vi "AudioTest.Parse SoundCheck Data Log TXT File.vi"(6 "Lim Center at Average(f), Float at center":bool, 8 "error in":errorcluster, 9 "Start_End":dbl[](array[numeric])=[500.0, 20000.0], 10 "Config Folder":path=path "C:/MTE/Audio Test/Config", 11 "SoundCheck Data File":path) -> (0 "error out":errorcluster, 1 "Meas Rslt":T3[](array[typedef]) {"Status" items=["LOG", "PASS", "FAIL", "ERROR"]}, 2 "Graph Names":string[](array[string]), 3 "Graphs":T5[](array[typedef]))   [LabVIEW 2018]
uses:
  TypeDefs/AudioTest.Analysis Data Record.ctl
  Common/Utils/Results/Result.Measurement Item.ctl
  Common/Utils/Results/Result.Measurement and Attribute Item Status.ctl
  TypeDefs/AudioTest.Graph Definitions.ctl
  TypeDefs/AudioTest.Result Plot Data.ctl
  Common/Utils/Errors/Error.Error Code List.ctl
  <vilib>/KATE/Files/File Utils.lvlib
panel:
  out "LimitPlots":T1[](array[typedef])
  out "Graph Defs":T2[](array[typedef])
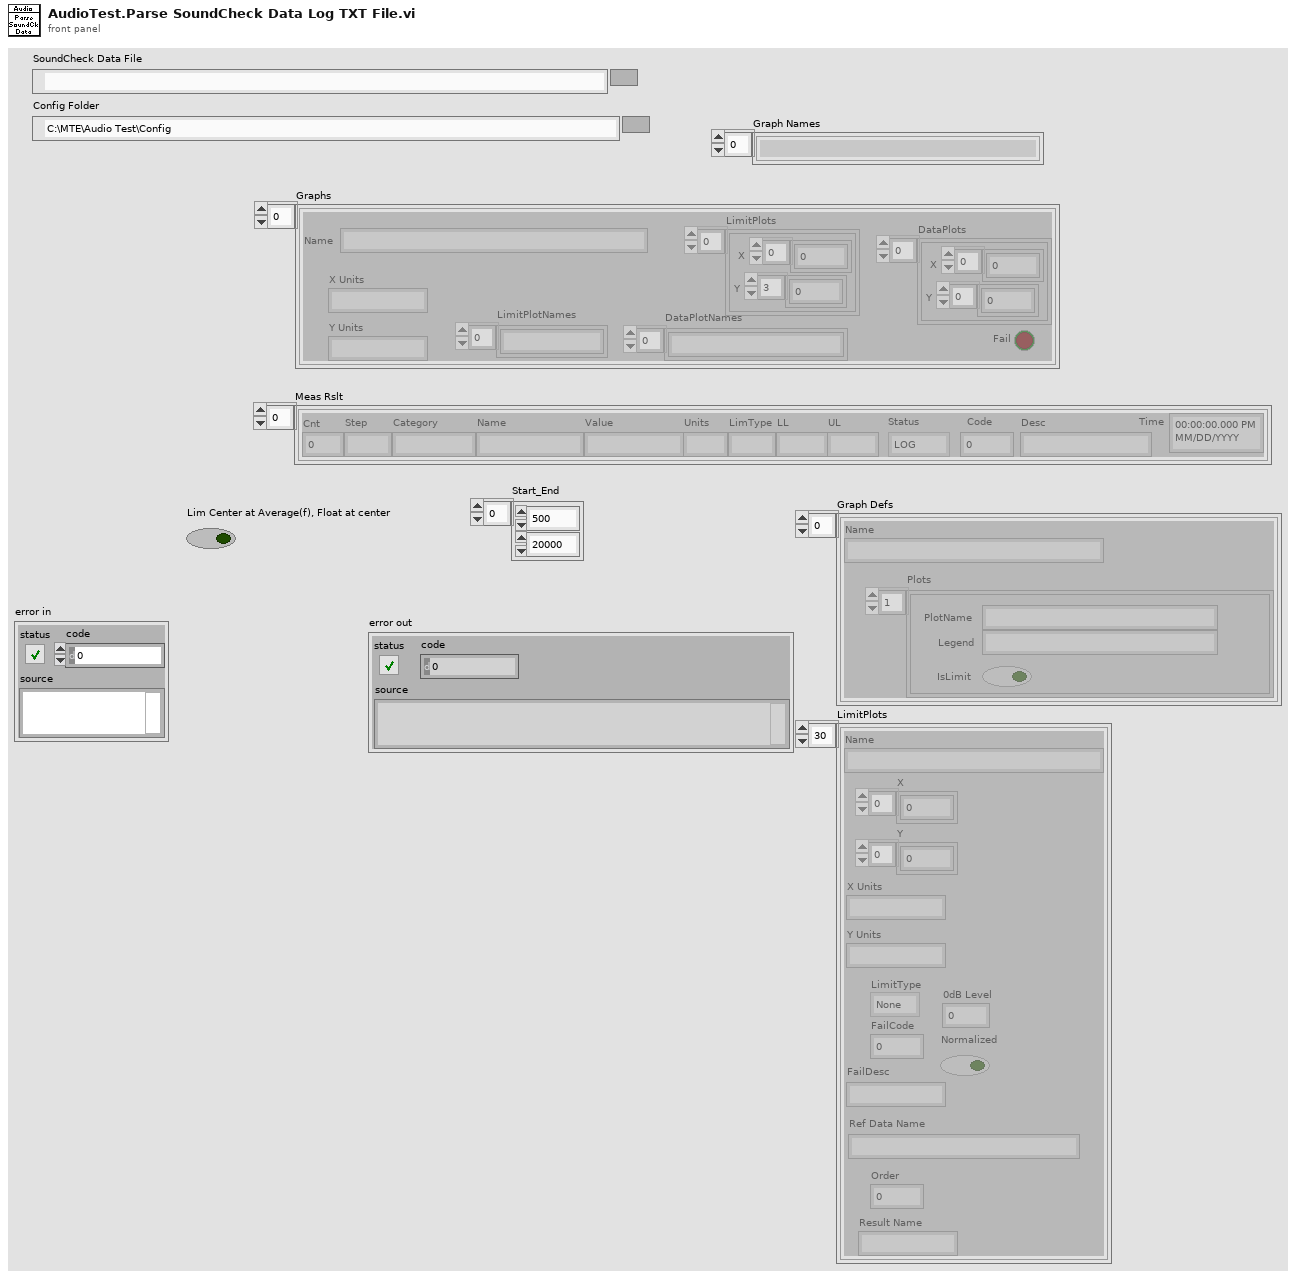
[diagram p1: front panel]
types:
  T1 = typedef "AudioTest.Result Plot Data.ctl" = cluster{"Order":i32, "Name":string, "X":dbl[], "Y":dbl[], "X Units":string, "Y Units":string, "LimitType":enum16{"None", "LL", "UL"}, "FailCode":i32, "FailDesc":string, "Ref Data Name":string, "Result Name":string, "0dB Level":dbl, "Normalized":bool}
  T2 = typedef "AudioTest.Graph Definitions.ctl" = cluster{"Name":string, "Plots":cluster{"PlotName":string, "Legend":string, "IsLimit":bool}[]}
  T3 = typedef "Result.Measurement Item.ctl" = cluster{"Cnt":i32, "Step":string, "Category":string, "Name":string, "Value":string, "Units":string, "LimType":string, "LL":string, "UL":string, "Status":T4, "Code":i32, "Desc":string, "Time":timestamp}
  T4 = typedef "Result.Measurement and Attribute Item Status.ctl" = i32
  T5 = typedef "AudioTest.Analysis Data Record.ctl" = cluster{"Name":string, "X Units":string, "Y Units":string, "DataPlots":cluster{"X":dbl[], "Y":dbl[]}[], "LimitPlots":cluster{"X":dbl[], "Y":dbl[]}[], "DataPlotNames":string[], "LimitPlotNames":string[], "Fail":bool}
  T6 = typedef "Error.Error Code List.ctl" = i32
  T7 = cluster{"Data":string, "Graphs":T5[], "Graph Names":string[], "RawPlots":T1[], "LimitPlots":T1[], "Meas Rslt":T3[], "PlotNames":variant, "Graph Defs":T2[]}
  T8 = cluster{"PlotName":string, "Legend":string, "IsLimit":bool}[]
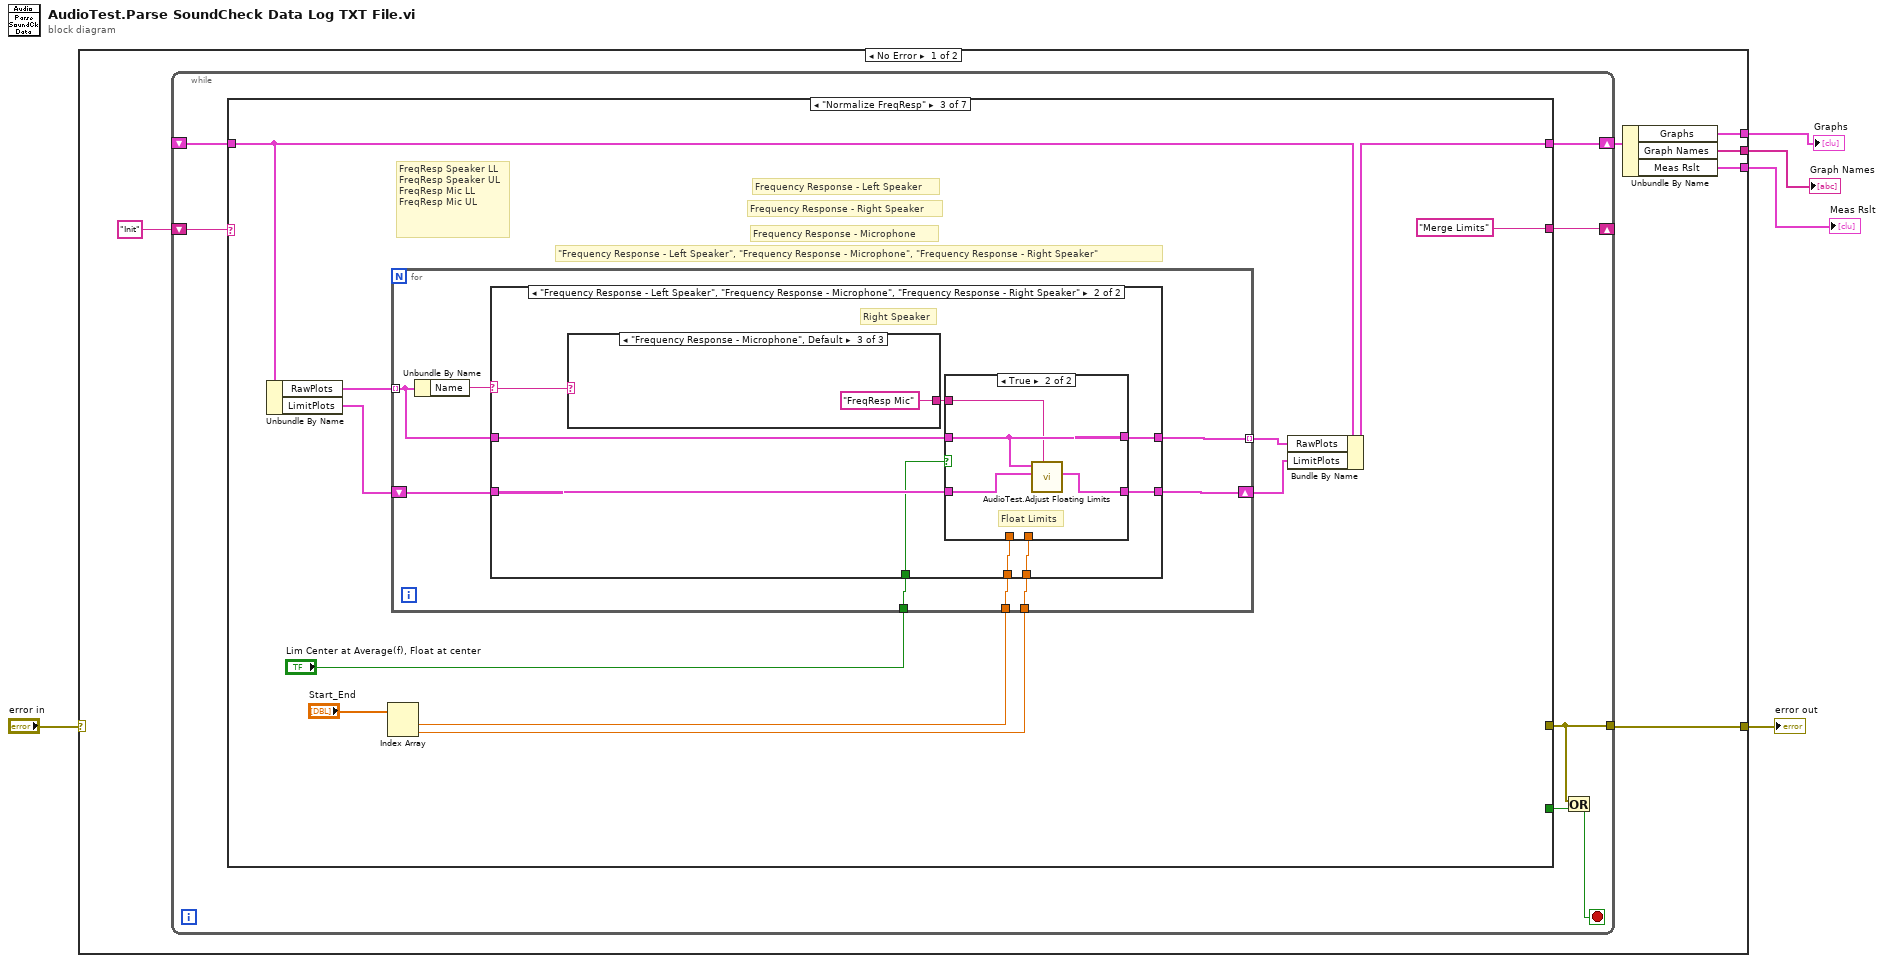
[diagram p0: block diagram]
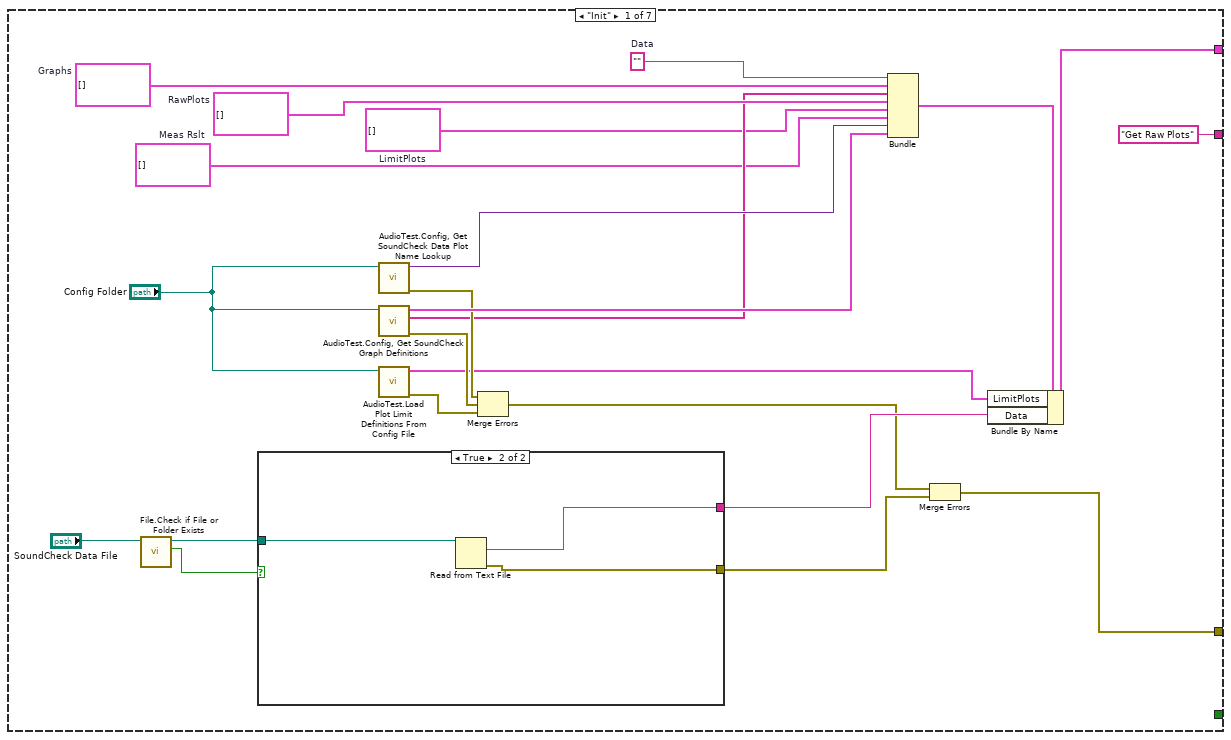
[diagram p2: hidden frame]
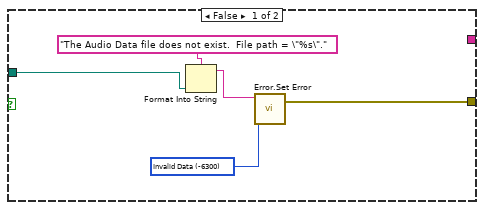
[diagram p3: hidden frame]
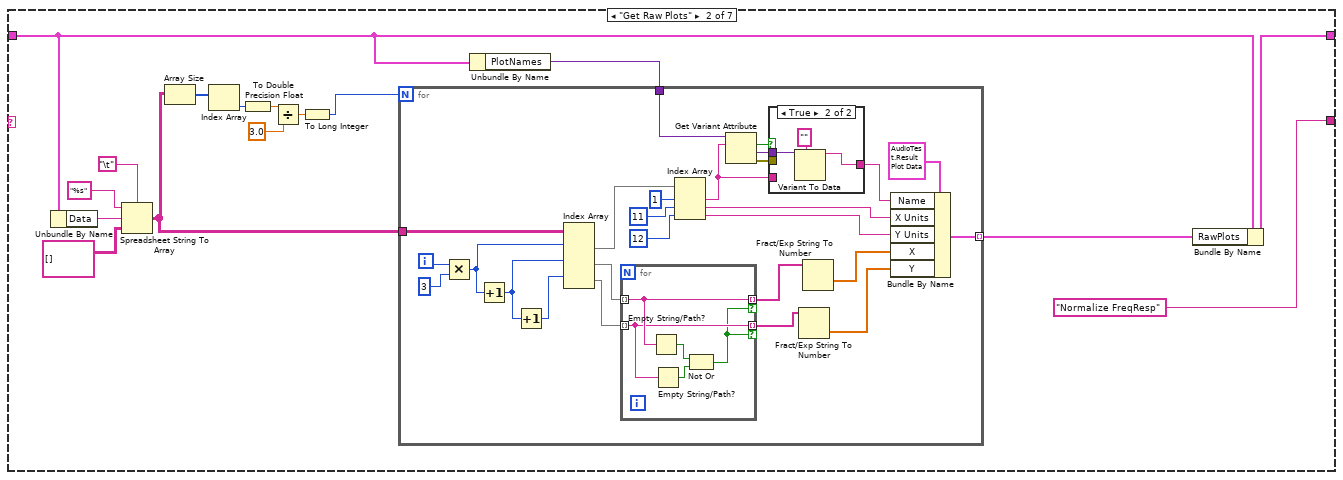
[diagram p4: hidden frame]
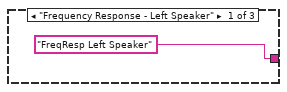
[diagram p7: hidden frame]
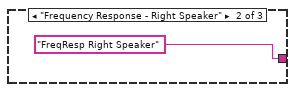
[diagram p8: hidden frame]
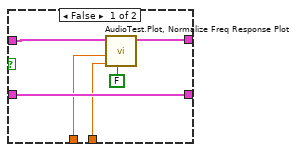
[diagram p9: hidden frame]
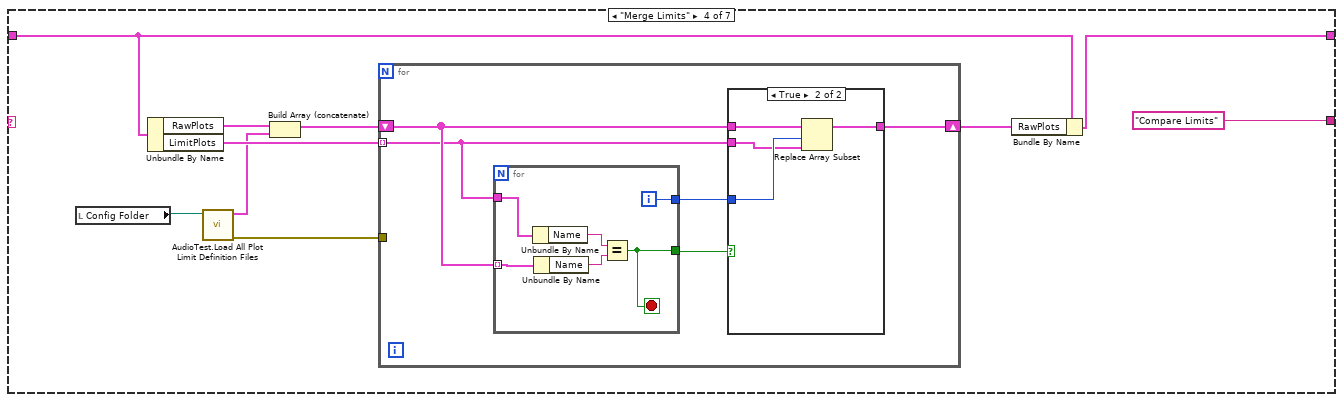
[diagram p10: hidden frame]
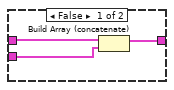
[diagram p11: hidden frame]
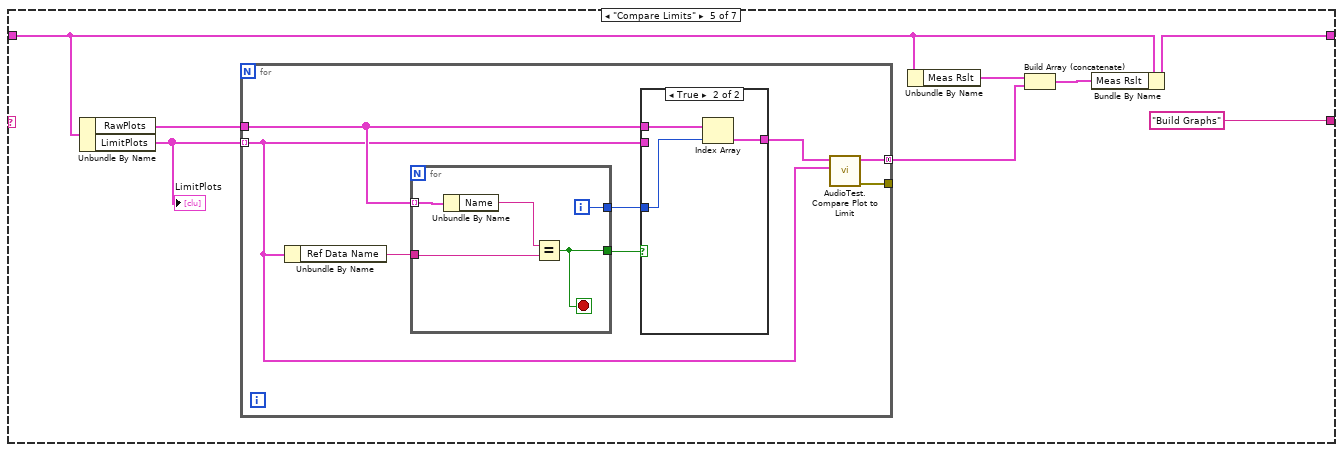
[diagram p12: hidden frame]
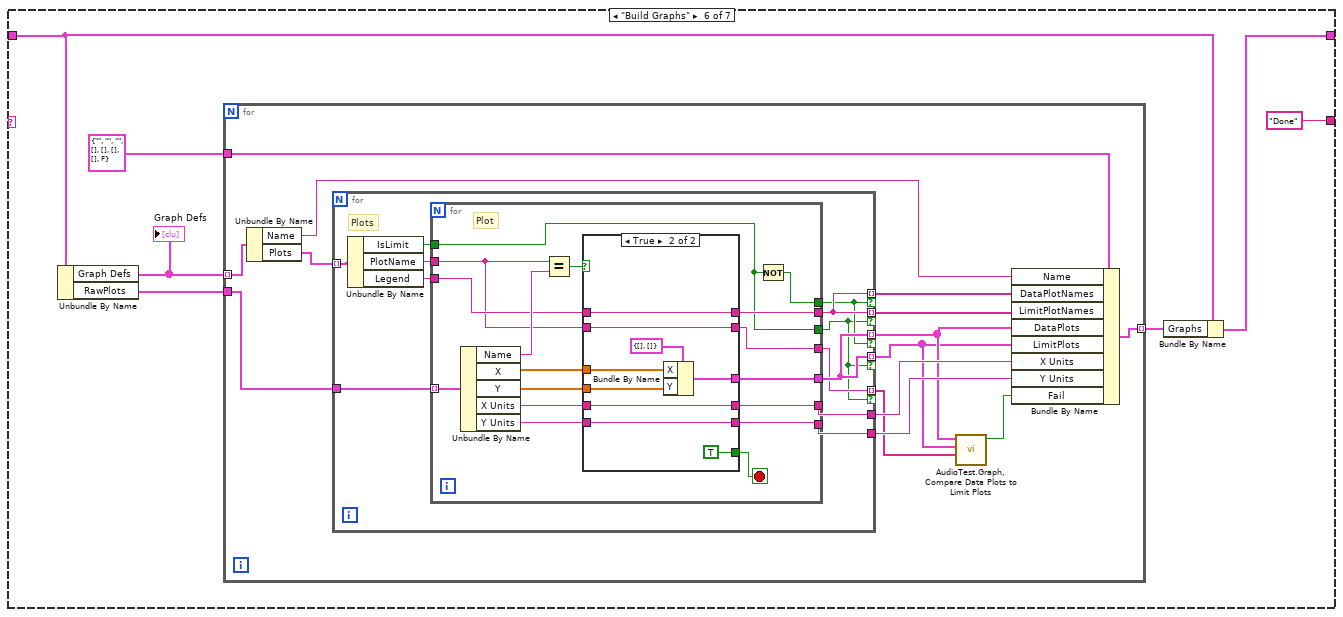
[diagram p14: hidden frame]
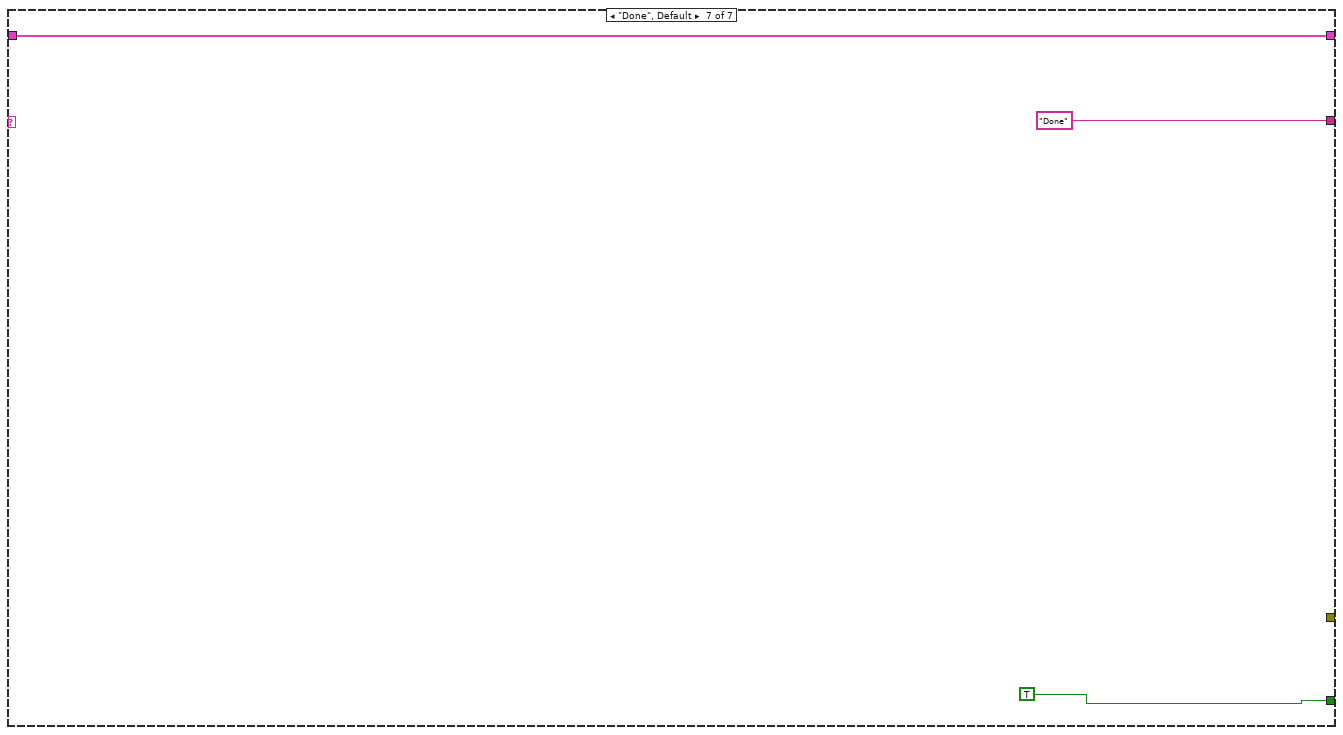
[diagram p16: hidden frame]
diagram:
  n1 = case shown="No Error" "error in" {
    selector: "error in" -> [_ w258]
    tunnel: [w10 w258] -> w5
    tunnel: [w8 _] -> w3
    tunnel: [w7 _] -> w2
    tunnel: [w6 _] -> w1
    frame No Error {
      n2 = while {
        shift-right: [w18] -> w9
        shift-left: _ -> [w12]
        tunnel: [w15] -> w10
        shift-right: [w16] -> _
        shift-left: "Init" -> [w17]
        stop <- w14 stop-if-true
        n3 = case shown="\"Normalize FreqResp\"" w17 {
          tunnel: [w34 w54 w109 w151 w177 w197 w255] -> w18
          tunnel: [w25 _ _ _ _ _ _] -> w15
          tunnel: ["Get Raw Plots" "Normalize FreqResp" "Merge Limits" "Compare Limits" "Build Graphs" "Done" "Done"] -> w16
          tunnel: [_ _ _ _ _ _ TRUE] -> w13
          tunnel: w12 -> [_ w51 w110 w152 w175 w198 w255]
          frame "Init" {
            w19 = T3[] []  # Meas Rslt
            w23 = T1[] []  # LimitPlots
            w32 = T1[] []  # RawPlots
            w36 = T5[] []  # Graphs
            w41 = ""  # Data
            n4 = call <vilib>:"File.Check if File or Folder Exists.vi"("Path"="SoundCheck Data File") -> ("Exists"=w39:bool, "Dup Path"=w38:path)  [unwired: 6 in, 3 out]
            n5 = case shown="True" w39 {
              tunnel: w38 -> [w44 w49]
              tunnel: [w42 w48] -> w26
              tunnel: [_ w47] -> w33
              frame False {
                w46 = T6 -6300 items=["No Error"=0, "Abort"=-2, "Misc"=-5000, "Fixture Error"=-5100, "File IO - General"=-5200, "FIle IO - Config Error"=-5201, "Instrument - General"=-5300, "Instrument - Serial Com"=-5301, "Instrument - Camera"=-5302, "Instrument - PS"=-5303, "Instrument - Oscilloscope"=-5304, "Instrument - Function Gen"=-5305, "Instrument - Load"=-5306, "Instrument - Meter"=-5307, "Instrument - Power Control"=-5308, "Instrument - Motion"=-5309, "Instrument - RF"=-5310, "System Exe"=-5400, "Image Processing"=-5500, "Communication"=-5600, "Script - Syntax Error"=-6000, "Script - Invalid Name or Param"=-6100, "Script - Timeout"=-6200, "Invalid Data"=-6300, "FW Update Error"=-6500] ("Std Code")
                n6 = Format Into String(format string="The Audio Data file does not exist.  File path = \"%s\"." ("Desc"), w44) -> (resulting string=w43:string)  [unwired: 2 in, 1 out]
                n7 = call "Error.Set Error.vi"("Code"=w46, "Desc"=w43) -> ("error out"=w42:errorcluster)  [unwired: 5 in]
              }
              frame True {
                n8 = Read from Text File(file (use dialog)=w49) -> (text=w47:string, error out=w48:errorcluster)  [unwired: 3 in, 2 out]
              }
            }
            n9 = call "AudioTest.Config, Get SoundCheck Data Plot Name Lookup.vi"("Config Folder"="Config Folder") -> ("error out"=w29:errorcluster, "PlotNames"=w31:variant)  [unwired: 9 in]
            n10 = call "AudioTest.Config, Get SoundCheck Graph Definitions.vi"("Config Folder"="Config Folder") -> ("error out"=w28:errorcluster, "Graph Names"=w24:string[], "Graph Defs"=w30:T2[])  [unwired: 8 in]
            n11 = call "AudioTest.Load Plot Limit Definitions From Config File.vi"("Config Folder"="Config Folder") -> ("error out"=w20:errorcluster, "LimitPlots"=w21:T1[])  [unwired: 9 in]
            n12 = Merge Errors(w29, w28, w20) -> (w27:errorcluster)
            n13 = Bundle("Data"=w41, "Graphs"=w36, "Graph Names"=w24, "RawPlots"=w32, "LimitPlots"=w23, "Meas Rslt"=w19, "PlotNames"=w31, "Graph Defs"=w30) -> (w35:T7)  [unwired: 1 in]
            n14 = Merge Errors(w27, w26) -> (w25:errorcluster)
            n15 = Bundle By Name(cluster=w35, "LimitPlots"=w21, "Data"=w33) -> (w34:T7)
          }
          frame "Get Raw Plots" {
            n16 = Unbundle By Name(w51) -> ("Data"=w64:string)
            n17 = Spreadsheet String To Array(delimiter (Tab)="\t", format string="%s", spreadsheet string=w64, array type (2D Dbl)=string[][] []) -> (array=w55:string[][])
            n18 = Array Size(array=w55) -> (size(s)=w60:i32[])
            n19 = Index Array(array=w60) -> (element=w59:i32)  [unwired: 1 in]
            n20 = To Double Precision Float(number=w59) -> (double precision float=w58:dbl)
            n21 = Divide(x=w58, y=3.0) -> (x/y=w56:dbl)
            n22 = To Long Integer(number=w56) -> (32bit integer=w52:i32)
            n23 = Unbundle By Name(w51) -> ("PlotNames"=w50:variant)
            n24 = for {
              N: w52 -> [_]
              tunnel: w55 -> [w91]
              tunnel: [w79] -> w53 mode=indexing
              tunnel: w50 -> [w72]
              i -> [w90]
              n25 = Multiply(x=w90, y=3) -> (x*y=w88:i32)
              n26 = Increment(x=w88) -> (x+1=w87:i32)
              n27 = Increment(x=w87) -> (x+1=w86:i32)
              n28 = Index Array(array=w91, index (row) #1=w88, index (row) #2=w87, index (row) #3=w86) -> (element #1=w85:string[], element #2=w76:string[], element #3=w75:string[])  [unwired: 3 in]
              n29 = for {
                tunnel: w76 -> [w98] mode=indexing
                tunnel: w75 -> [w97] mode=indexing
                tunnel: [w98] -> w74 mode=indexing if=w96
                tunnel: [w97] -> w73 mode=indexing if=w96
                n30 = Empty String/Path?(string/path=w98) -> (empty?=w100:bool)
                n31 = Empty String/Path?(string/path=w97) -> (empty?=w99:bool)
                n32 = Not Or(1:w99, 2:w100) -> (0:w96:bool)
              }
              n33 = Index Array(array=w85, index #1=1 ("index"), index #2=11 ("index"), index #3=12 ("index")) -> (element #1=w66:string, element #2=w71:string, element #3=w80:string)
              n34 = Get Variant Attribute(Variant=w72, name=w66) -> (found=w70:bool, value=w69:variant, error out=w68:errorcluster)  [unwired: 2 in, 1 out]
              n35 = case shown="True" w70 {
                tunnel: w69 -> [_ w95]
                tunnel: w68 -> [_ _]
                tunnel: [w92 w93] -> w67
                tunnel: w66 -> [w92 _]
                frame False {
                }
                frame True {
                  n36 = Variant To Data(type="", Variant=w95) -> (data=w93:string)  [unwired: 1 in, 1 out]
                }
              }
              n37 = Fract/Exp String To Number(string=w73) -> (number=w77:dbl[])  [unwired: 3 in, 1 out]
              n38 = Fract/Exp String To Number(string=w74) -> (number=w78:dbl[])  [unwired: 3 in, 1 out]
              n39 = Bundle By Name(cluster=T1 {"Order"=0, "Name"="", "X"=[], "Y"=[], "X Units"="", "Y Units"="", "LimitType"=enum."None", "FailCode"=0, "FailDesc"="", "Ref Data Name"="", "Result Name"="", "0dB Level"=0.0, "Normalized"=FALSE}, "Name"=w67, "X Units"=w71, "Y Units"=w80, "X"=w78, "Y"=w77) -> (w79:T1)
            }
            n40 = Bundle By Name(cluster=w51, "RawPlots"=w53) -> (w54:T7)
          }
          frame "Normalize FreqResp" {
            # "\"Frequency Response - Left Speaker\", \"Frequency Response - Microphone\", \"Frequency Response - Right Speaker\""
            # "FreqResp Speaker LL\nFreqResp Speaker UL\nFreqResp Mic LL\nFreqResp Mic UL"
            # "Frequency Response - Right Speaker"
            # "Frequency Response - Microphone"
            # "Frequency Response - Left Speaker"
            n41 = Unbundle By Name(w110) -> ("RawPlots"=w105:T1[], "LimitPlots"=w103:T1[])
            n42 = Index Array(array="Start_End") -> (element #1=w107:dbl, element #2=w106:dbl)  [unwired: 2 in]
            n43 = for {
              tunnel: w105 -> [w118] mode=indexing
              tunnel: [w117] -> w102 mode=indexing
              shift-right: [w115] -> w101
              shift-left: w103 -> [w116]
              tunnel: "Lim Center at Average(f), Float at center" -> [w114]
              tunnel: w107 -> [w113]
              tunnel: w106 -> [w112]
              n44 = Unbundle By Name(w118) -> ("Name"=w119:string)
              n45 = case shown="\"Frequency Response - Left Speaker\", \"Frequency Response - Microphone\", \"Frequency Response - Right Speaker\"" w119 {
                selector: w119 -> [_ w122]
                tunnel: w118 -> [w121 w130]
                tunnel: [w121 w129] -> w117
                tunnel: w116 -> [w120 w128]
                tunnel: [w120 w127] -> w115
                tunnel: w114 -> [_ w126]
                tunnel: w113 -> [_ w125]
                tunnel: w112 -> [_ w124]
                frame Default {
                }
                frame "Frequency Response - Left Speaker", "Frequency Response - Microphone", "Frequency Response - Right Speaker" {
                  # "Right Speaker"
                  n46 = case shown="\"Frequency Response - Microphone\", Default" w122 {
                    tunnel: ["FreqResp Left Speaker" ("regular expression") "FreqResp Right Speaker" ("regular expression") "FreqResp Mic" ("regular expression")] -> w123
                    frame "Frequency Response - Left Speaker" {
                    }
                    frame "Frequency Response - Right Speaker" {
                    }
                    frame "Frequency Response - Microphone", Default {
                    }
                  }
                  n47 = case shown="True" w126 {
                    tunnel: w130 -> [w139 w143]
                    tunnel: [w138 w143] -> w129
                    tunnel: w128 -> [w137 w142]
                    tunnel: [w137 w141] -> w127
                    tunnel: w125 -> [w136 _]
                    tunnel: w124 -> [w135 _]
                    tunnel: w123 -> [_ w140]
                    frame False {
                      n48 = call "AudioTest.Plot, Normalize Freq Response Plot.vi"("Average(F), Center_Min_Max(T)"=FALSE, "F End"=w135, "F Start"=w136, "Data In"=w139) -> ("Data Out"=w138:T1)  [unwired: 6 in, 1 out]
                    }
                    frame True {
                      # "Float Limits"
                      n49 = call "AudioTest.Adjust Floating Limits.vi"("Lim Name"=w140, "LimitPlots"=w142, "Plot"=w143) -> ("LimitPlots Out"=w141:T1[])  [unwired: 8 in]
                    }
                  }
                }
              }
            }
            n50 = Bundle By Name(cluster=w110, "RawPlots"=w102, "LimitPlots"=w101) -> (w109:T7)
          }
          frame "Merge Limits" {
            n51 = local read "Config Folder"() -> (w150:path)
            n52 = Unbundle By Name(w152) -> ("RawPlots"=w147:T1[], "LimitPlots"=w145:T1[])
            n53 = call "AudioTest.Load All Plot Limit Definition Files.vi"("Config Folder"=w150) -> ("error out"=w149:errorcluster, "LimitPlots"=w144:T1[])  [unwired: 9 in]
            n54 = Build Array (concatenate)(w147, w144) -> (w148:T1[])
            n55 = for {
              tunnel: w145 -> [w155] mode=indexing
              shift-right: [w154] -> w146
              shift-left: w148 -> [w156]
              tunnel: w149 -> [_]
              n56 = for {
                tunnel: w156 -> [w170] mode=indexing
                tunnel: w155 -> [w171]
                tunnel: [w167] -> w158
                tunnel: [w166] -> w157
                i -> [w166]
                stop <- w167 stop-if-true
                n57 = Unbundle By Name(w171) -> ("Name"=w169:string)
                n58 = Unbundle By Name(w170) -> ("Name"=w168:string)
                n59 = Equal?(x=w169, y=w168) -> (x = y?=w167:bool)
              }
              n60 = case shown="True" w158 {
                tunnel: w157 -> [_ w164]
                tunnel: w156 -> [w161 w165]
                tunnel: w155 -> [w159 w163]
                tunnel: [w160 w162] -> w154
                frame False {
                  n61 = Build Array (concatenate)(w161, w159) -> (w160:T1[])
                }
                frame True {
                  n62 = Replace Array Subset(array=w165, new element=w163, index=w164) -> (w162:T1[])
                }
              }
            }
            n63 = Bundle By Name(cluster=w152, "RawPlots"=w146) -> (w151:T7)
          }
          frame "Compare Limits" {
            n64 = Unbundle By Name(w175) -> ("RawPlots"=w176:T1[], "LimitPlots"=w178:T1[])
            "LimitPlots" <- w178
            n65 = for {
              tunnel: w178 -> [w182] mode=indexing
              tunnel: w176 -> [w185]
              tunnel: [w181] -> w172 mode=concatenating
              tunnel: [w180] -> _
              n66 = Unbundle By Name(w182) -> ("Ref Data Name"=w184:string)
              n67 = for {
                tunnel: w185 -> [w195] mode=indexing
                tunnel: [w194] -> w187
                tunnel: [w193] -> w186
                tunnel: w184 -> [w191]
                i -> [w193]
                stop <- w194 stop-if-true
                n68 = Unbundle By Name(w195) -> ("Name"=w192:string)
                n69 = Equal?(x=w192, y=w191) -> (x = y?=w194:bool)
              }
              n70 = case shown="True" w187 {
                tunnel: w186 -> [_ w189]
                tunnel: w185 -> [_ w190]
                tunnel: w182 -> [_ _]
                tunnel: [_ w188] -> w183
                frame False {
                }
                frame True {
                  n71 = Index Array(array=w190, index=w189) -> (element=w188:T1)
                }
              }
              n72 = call "AudioTest.Compare Plot to Limit.vi"("Plot Limit"=w182, "Plot Data"=w183) -> ("error out"=w180:errorcluster, "Meas Rslt"=w181:T3[])  [unwired: 6 in, 2 out]
            }
            n73 = Unbundle By Name(w175) -> ("Meas Rslt"=w174:T3[])
            n74 = Build Array (concatenate)(w174, w172) -> (w173:T3[])
            n75 = Bundle By Name(cluster=w175, "Meas Rslt"=w173) -> (w177:T7)
          }
          frame "Build Graphs" {
            n76 = Unbundle By Name(w198) -> ("Graph Defs"=w202:T2[], "RawPlots"=w196:T1[])
            "Graph Defs" <- w202
            n77 = for {
              tunnel: w202 -> [w216] mode=indexing
              tunnel: w196 -> [w214]
              tunnel: T5 {"Name"="", "X Units"="", "Y Units"="", "DataPlots"=[], "LimitPlots"=[], "DataPlotNames"=[], "LimitPlotNames"=[], "Fail"=FALSE} -> [w213]
              tunnel: [w207] -> w199 mode=indexing
              n78 = Unbundle By Name(w216) -> ("Name"=w212:string, "Plots"=w215:T8)
              n79 = for {
                tunnel: w215 -> [w227] mode=indexing
                tunnel: w214 -> [w228]
                tunnel: [w224] -> w210
                tunnel: [w223] -> w211
                tunnel: [w222] -> w209 mode=indexing if=w217
                tunnel: [w222] -> w208 mode=indexing if=w219
                tunnel: [w220] -> w206 mode=indexing if=w219
                tunnel: [w220] -> w205 mode=indexing if=w217
                tunnel: [w218] -> w204 mode=indexing if=w217
                # "Plots"
                n80 = Unbundle By Name(w227) -> ("IsLimit"=w221:bool, "PlotName"=w226:string, "Legend"=w225:string)
                n81 = for {
                  tunnel: w228 -> [w245] mode=indexing
                  tunnel: w226 -> [w230]
                  tunnel: w225 -> [w234]
                  tunnel: [w238] -> w220
                  tunnel: [w236] -> w224
                  tunnel: [w235] -> w223
                  tunnel: [w233] -> w222
                  tunnel: [w231] -> w217
                  tunnel: w221 -> [w231]
                  tunnel: [w232] -> w219
                  tunnel: [w229] -> w218
                  stop <- w237 stop-if-true
                  # "Plot"
                  n82 = Unbundle By Name(w245) -> ("Name"=w244:string, "X"=w240:dbl[], "Y"=w239:dbl[], "X Units"=w242:string, "Y Units"=w241:string)
                  n83 = Equal?(x=w230, y=w244) -> (x = y?=w243:bool)
                  n84 = case shown="True" w243 {
                    tunnel: w242 -> [_ w249]
                    tunnel: w241 -> [_ w248]
                    tunnel: w240 -> [_ w253]
                    tunnel: w239 -> [_ w252]
                    tunnel: [_ w251] -> w238
                    tunnel: [_ TRUE] -> w237
                    tunnel: [_ w249] -> w236
                    tunnel: [_ w248] -> w235
                    tunnel: w234 -> [_ w247]
                    tunnel: [_ w247] -> w233
                    tunnel: [_ w246] -> w229
                    tunnel: w230 -> [_ w246]
                    frame False {
                    }
                    frame True {
                      n85 = Bundle By Name(cluster=cluster{"X":dbl[], "Y":dbl[]} {"X"=[], "Y"=[]} ("Plot"), "X"=w253, "Y"=w252) -> (w251:cluster{"X":dbl[], "Y":dbl[]})
                    }
                  }
                  n86 = Not(x=w231) -> (.not. x?=w232:bool)
                }
              }
              n87 = call "AudioTest.Graph, Compare Data Plots to Limit Plots.vi"("Limit Names"=w204, "Limits"=w205, "Data"=w206) -> ("FAIL"=w203:bool)  [unwired: 8 in]
              n88 = Bundle By Name(cluster=w213, "Name"=w212, "DataPlotNames"=w208, "LimitPlotNames"=w209, "DataPlots"=w206, "LimitPlots"=w205, "X Units"=w210, "Y Units"=w211, "Fail"=w203) -> (w207:T5)
            }
            n89 = Bundle By Name(cluster=w198, "Graphs"=w199) -> (w197:T7)
          }
          frame "Done", Default {
          }
        }
        n90 = Or(x=w15, y=w13) -> (x .or. y?=w14:bool)
      }
      n91 = Unbundle By Name(w9) -> ("Graphs"=w8:T5[], "Graph Names"=w7:string[], "Meas Rslt"=w6:T3[])
    }
    frame Error {
    }
  }
  "error out" <- w5
  "Graphs" <- w3
  "Graph Names" <- w2
  "Meas Rslt" <- w1
